vi "DriveDisplacement.vi"(8 "Error In":errorcluster, 11 "Boolean":bool) -> (0 "Error Out":errorcluster)   [LabVIEW 2017]
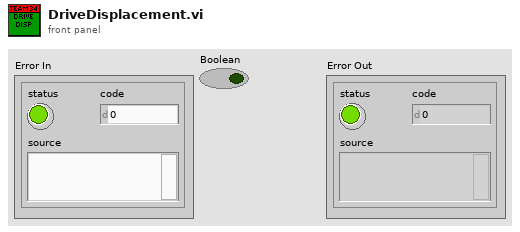
[diagram p1: front panel]
types:
  T1 = cluster{"Velocity X":dbl, "Velocity Y":dbl, "Velocity Z":dbl, "Displacement X":dbl, "Displacement Y":dbl, "Displacement Z":dbl}
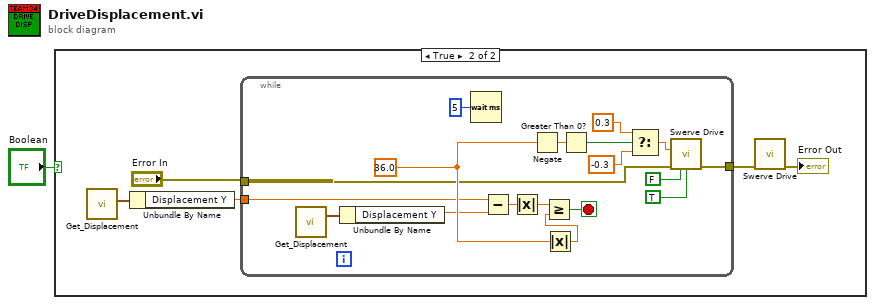
[diagram p0: block diagram]
diagram:
  n1 = case shown="True" "Boolean" {
    frame False {
    }
    frame True {
      n2 = call <vilib>:"Get_Displacement.vi"() -> ("Displacement"=w6:T1)  [unwired: 11 in]
      n3 = Unbundle By Name(w6) -> ("Displacement Y"=w4:dbl)
      n4 = while {
        tunnel: [w21] -> w5
        tunnel: w4 -> [w10]
        tunnel: "Error In" -> [w9]
        stop <- w22 stop-if-true
        w11 = 36.0 ("Distance to Drive")
        n5 = call <vilib>:"Get_Displacement.vi"() -> ("Displacement"=w8:T1)  [unwired: 11 in]
        n6 = Unbundle By Name(w8) -> ("Displacement Y"=w7:dbl)
        n7 = Wait (ms)(milliseconds to wait=u32 5) -> ()  [unwired: 1 out]
        n8 = Subtract(x=w10, y=w7) -> (x-y=w24:dbl)
        n9 = Absolute Value(x=w24) -> (abs(x)=w23:dbl)
        n10 = Negate(x=w11) -> (-x=w12:dbl)
        n11 = Absolute Value(x=w11) -> (abs(x)=w13:dbl)
        n12 = Greater Or Equal?(x=w23, y=w13) -> (x >= y?=w22:bool)
        n13 = Greater Than 0?(x=w12) -> (x > 0?=w16:bool)
        n14 = Select(t=0.3 ("X"), s=w16, f=-0.3 ("X")) -> (s? t:f=w15:dbl)
        n15 = call "Swerve Drive.vi"("Y"=w15, "Error In"=w9, "Robot Centric?"=FALSE, "Autonomous?"=TRUE) -> ("Error Out"=w21:errorcluster)  [unwired: 7 in, 4 out]
      }
      n16 = call "Swerve Drive.vi"("Error In"=w5) -> ("Error Out"=→"Error Out":errorcluster)  [unwired: 10 in, 4 out]
    }
  }
